vi "CheckBfieldValue .vi"(6 "deadband":dbl=0.05 format="%#_13g", 7 "B [T] new":dbl, 11 "MagSpec_Bella in":refnum<class "MagSpec_Bella.lvclass">) -> (3 "MagSpec_Bella out":refnum<class "MagSpec_Bella.lvclass">, 5 "Same?":bool)   [LabVIEW 2013, in "MagSpec_Bella.lvclass"]
uses:
  MagSpec_Bella.lvclass
  MagSpec_Bella.lvclass/MagSpec_Bella.ctl
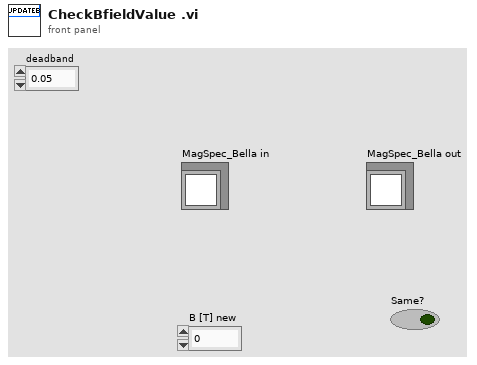
[diagram p1: front panel]
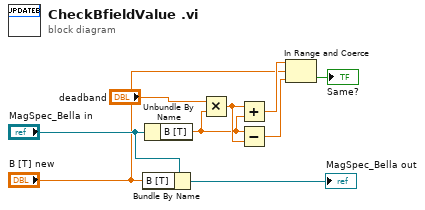
[diagram p0: block diagram]
diagram:
  n1 = Bundle By Name(cluster="MagSpec_Bella in", "B [T]"="B [T] new") -> (→"MagSpec_Bella out":refnum<class "MagSpec_Bella.lvclass">)
  n2 = Unbundle By Name("MagSpec_Bella in") -> ("B [T]"=w4:dbl)
  n3 = Multiply(x="deadband", y=w4) -> (x*y=w7:dbl)
  n4 = Add(x=w7, y=w4) -> (x+y=w6:dbl)
  n5 = Subtract(x=w4, y=w7) -> (x-y=w8:dbl)
  n6 = In Range and Coerce(upper limit=w6, x="B [T] new", lower limit=w8) -> (In Range?=→"Same?":bool)  [unwired: 1 out]
